vi "Sagar C V RLC (series) graph.vi"() -> ()   [LabVIEW 2021]
panel:
  in  "stop":bool
  out "XY Graph":cluster{"Y":dbl[], "Y":dbl[]}[](graph)
  out "Current":dbl
  out "Impedance":dbl
  out "XC":dbl
  out "XL":dbl
  in  "C(Capacitance)":dbl
  in  "R(Resistance)":dbl
  in  "Vin":dbl
  out "Frequency":dbl format="%#_13g"
  in  "L(Inductance)":dbl
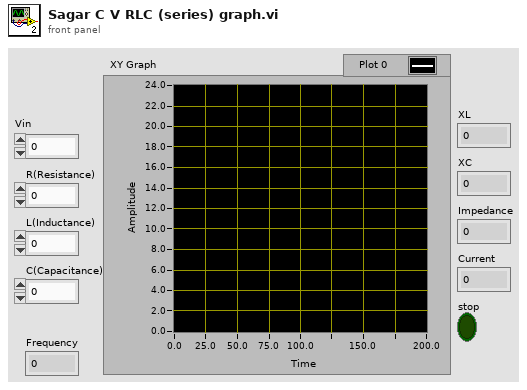
[diagram p1: front panel]
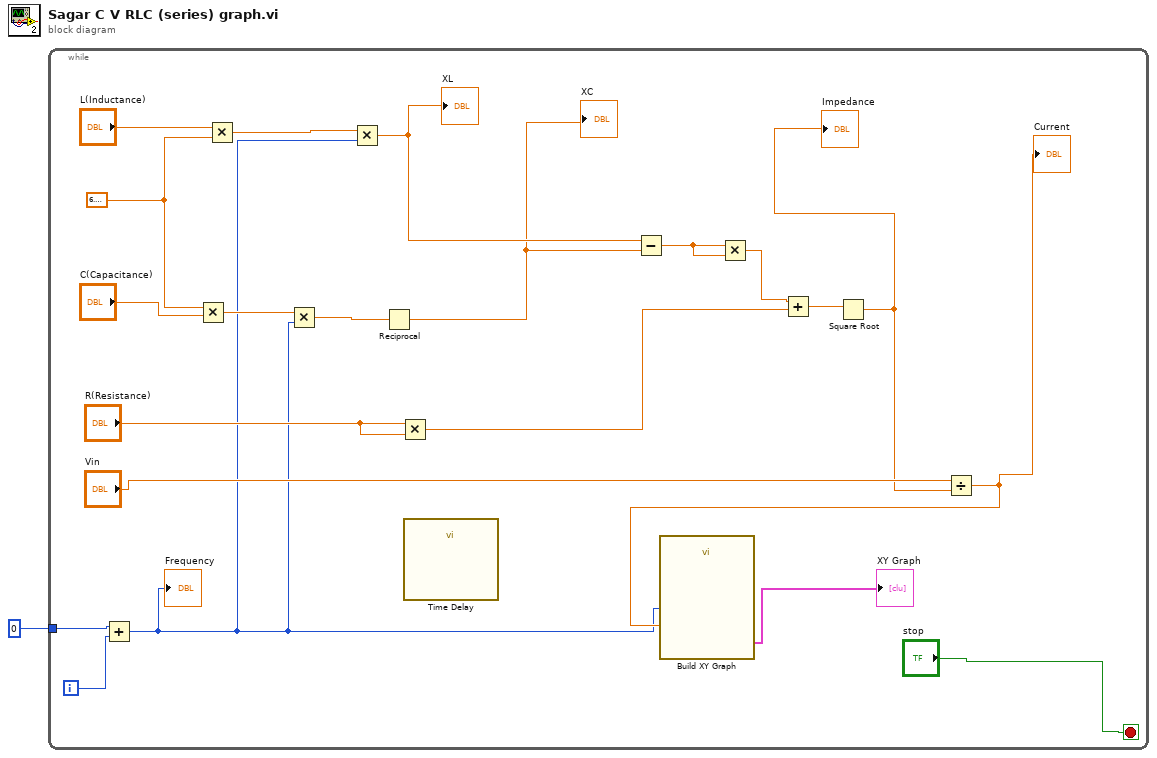
[diagram p0: block diagram]
diagram:
  n1 = while {
    tunnel: 0 -> [w2]
    i -> [w22]
    stop <- "stop" stop-if-true
    w18 = 6.283185307179586
    n2 = Add(x=w2, y=w22) -> (x+y=w5:i32)
    "Frequency" <- w5
    n3 = Multiply(x=w18, y="C(Capacitance)") -> (x*y=w17:dbl)
    n4 = Multiply(x="L(Inductance)", y=w18) -> (x*y=w19:dbl)
    n5 = Multiply(x=w17, y=w5) -> (x*y=w16:dbl)
    n6 = Multiply(x=w19, y=w5) -> (x*y=w14:dbl)
    "XL" <- w14
    n7 = Reciprocal(x=w16) -> (1/x=w13:dbl)
    "XC" <- w13
    n8 = Multiply(x="R(Resistance)", y="R(Resistance)") -> (x*y=w10:dbl)
    n9 = call "Time Delay"() -> ()  [unwired: 11 in, 1 out]
    n10 = Subtract(x=w14, y=w13) -> (x-y=w12:dbl)
    n11 = Multiply(x=w12, y=w12) -> (x*y=w11:dbl)
    n12 = Add(x=w11, y=w10) -> (x+y=w9:dbl)
    n13 = Square Root(x=w9) -> (sqrt(x)=w7:dbl)
    "Impedance" <- w7
    n14 = Divide(x="Vin", y=w7) -> (x/y=w6:dbl)
    "Current" <- w6
    n15 = call "Build XY Graph"("Y Input"=w6, "X Input"=w5) -> ("XY Graph"=→"XY Graph":cluster{"X":dbl[], "Y":dbl[]}[])  [unwired: 8 in, 1 out]
  }
